vi "PSK_Packet_Transmit.vi"() -> ()   [LabVIEW 2014]
uses:
  <vilib>/Waveform/DWDTOps.llb/DWDT Analog to Digital.vi
  <vilib>/Waveform/DWDTOps.llb/DWDT Digital to Binary U8.vi
  <instrlib>/niUSRP/niUSRP Write Tx Data (CDB Cluster).vi
  <vilib>/Waveform/DWDTOps.llb/DWDT Binary U8 to Digital.vi
  <vilib>/Waveform/DWDTOps.llb/DWDT Digital to Analog.vi
  <vilib>/measure/NI_MABase.lvlib
panel:
  out "Array":i8[][](array[numeric])
  out "Waveform Graph":waveform(dbl)(graph)
  in  "phase":dbl format="%.2p"
  in  "sampling info":cluster{"Fs":dbl, "#s":dbl}={"Fs"=1000.0, "#s"=1000.0} {"Fs" format="%.2p"}
  out "error out":errorcluster
  in  "stop":bool
  in  "USRP IP address":refnum<k15>="192.168.10.2"
  in  "Tx Parameters":T1={"Tx IQ Sampling\nRate [s/sec]"=400000.0, "Tx Frequency [Hz]"=915000000.0, "Tx Gain [dB]"=0.0, "Tx Antenna"="TX1"} {"Tx Gain [dB]" format="%#.6p"; "Tx Frequency [Hz]" format="%#.6p"; "Tx IQ Sampling\nRate [s/sec]" format="%#.6p"}
  out "Actual Tx Parameters":T1={"Tx IQ Sampling\nRate [s/sec]"=400000.0, "Tx Frequency [Hz]"=915000000.0, "Tx Gain [dB]"=0.0, "Tx Antenna"="TX1"} {"Tx Gain [dB]" format="%#.6p"; "Tx Frequency [Hz]" format="%#.6p"; "Tx IQ Sampling\nRate [s/sec]" format="%#.6p"}
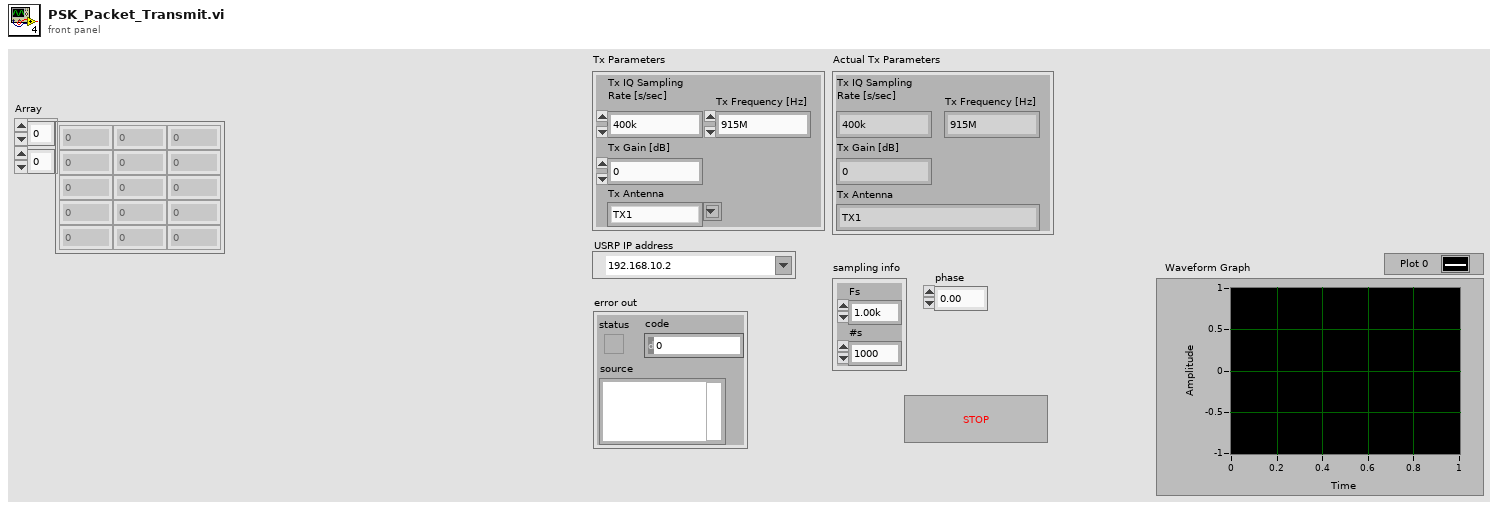
[diagram p1: front panel]
types:
  T1 = cluster{"Tx IQ Sampling\nRate [s/sec]":dbl, "Tx Frequency [Hz]":dbl, "Tx Gain [dB]":dbl, "Tx Antenna":string}
  T2 = typedef "niAMT.lvlib/Complex Data Waveform.ctl" = cluster{"t0":dbl, "dt":dbl, "Y":cdb[]}
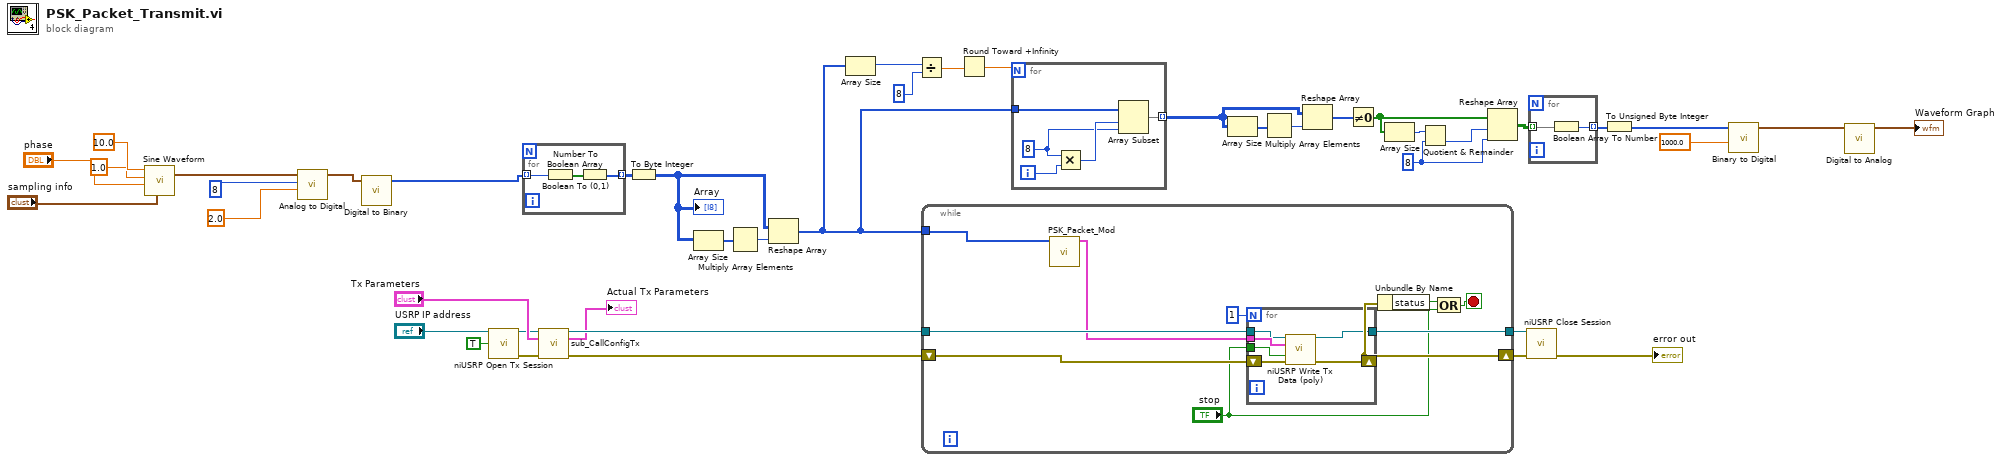
[diagram p0: block diagram]
diagram:
  w9 = 8 ("dimension size")
  n1 = call <vilib>:"Sine Waveform.vi"("sampling info"="sampling info", "phase"="phase", "amplitude"=1.0, "frequency"=10.0) -> ("signal out"=w32:waveform(dbl))  [unwired: 6 in, 1 out]
  n2 = call-poly <vilib>:"Analog to Digital.vi"("full-scale range (pk-pk)"=2.0, "resolution (16 bit)"=8, "analog waveform"=w32) -> ("digital waveform"=w25:digitalwaveform)  [unwired: 5 in, 3 out]
  n3 = call-poly <vilib>:"Digital to Binary.vi"("digital waveform"=w25) -> ("binary array"=w17:u8[])  [unwired: 9 in, 1 out]
  n4 = call <instrlib>:"niUSRP Open Tx Session.vi"("device names"="USRP IP address", "reset"=TRUE) -> ("session handle out"=w42:refnum<k15>, "error out"=w41:errorcluster)  [unwired: 12 in]
  n5 = for {
    tunnel: w17 -> [w46] mode=indexing
    tunnel: [w44] -> w21 mode=indexing
    n6 = Number To Boolean Array(number=w46) -> (Boolean array=w45:bool[])
    n7 = Boolean To (0,1)(Boolean=w45) -> (0, 1=w44:i16[])
  }
  n8 = call "sub_CallConfigTx.vi"("session handle"=w42, "Tx Parameters"="Tx Parameters", "error in"=w41) -> ("session handle out"=w36:refnum<k15>, "Actual Tx Parameters"=→"Actual Tx Parameters":T1, "error out"=w35:errorcluster)  [unwired: 10 in]
  n9 = To Byte Integer(number=w21) -> (8bit integer=w18:i8[][])
  "Array" <- w18
  n10 = Array Size(array=w18) -> (size(s)=w20:i32[])
  n11 = Multiply Array Elements(1:w20) -> (0:w19:i32)
  n12 = Reshape Array(w18, w19) -> (w12:i8[])
  n13 = Array Size(array=w12) -> (size(s)=w15:i32)
  n14 = Divide(x=w15, y=8) -> (x/y=w14:dbl)
  n15 = while {
    tunnel: w36 -> [w55]
    shift-right: [w52] -> w38
    shift-left: w35 -> [w56]
    tunnel: [w54] -> w37
    tunnel: w12 -> [w47]
    stop <- w51 stop-if-true
    n16 = call "PSK_Packet_Mod.vi"("user base bit pattern"=w47) -> ("output complex waveform"=w48:T2)  [unwired: 10 in]
    n17 = for {
      N: 1 -> [_]
      tunnel: w48 -> [w61]
      tunnel: w55 -> [w60]
      tunnel: [w59] -> w54
      tunnel: "stop" -> [w58]
      shift-right: [w57] -> w52
      shift-left: w56 -> [w62]
      n18 = call-poly <instrlib>:"niUSRP Write Tx Data (poly).vi"("session handle"=w60, "data"=w61, "end of data?"=w58, "error in (no error)"=w62) -> ("session handle out"=w59:refnum<k15>, "error out"=w57:errorcluster)  [unwired: 10 in]
    }
    n19 = Unbundle By Name(w52) -> ("status"=w53:bool)
    n20 = Compound Arithmetic op=OR(w53, "stop") -> (w51:bool)
  }
  n21 = Round Toward +Infinity(x=w14) -> (ceil(x): smallest int >= x=w13:dbl)
  n22 = for {
    N: w13 -> [_]
    tunnel: w12 -> [w67]
    tunnel: [w63] -> w1 mode=indexing
    i -> [w66]
    w64 = 8 ("x")
    n23 = Multiply(x=w64, y=w66) -> (x*y=w65:i32)
    n24 = Array Subset(array=w67, index=w65, length=w64) -> (w63:i8[])
  }
  n25 = Array Size(array=w1) -> (size(s)=w3:i32[])
  n26 = Multiply Array Elements(1:w3) -> (0:w4:i32)
  n27 = Reshape Array(w1, w4) -> (w2:i8[])
  n28 = Not Equal To 0?(x=w2) -> (x != 0?=w7:bool[])
  n29 = Array Size(array=w7) -> (size(s)=w8:i32)
  n30 = Quotient & Remainder(x=w8, y=w9) -> (floor(x/y)=w6:i32)  [unwired: 1 out]
  n31 = Reshape Array(w7, w6, w9) -> (w10:bool[][])
  n32 = call <instrlib>:"niUSRP Close Session.vi"("session handle"=w37, "error in (no error)"=w38) -> ("error out"=→"error out":errorcluster)  [unwired: 13 in]
  n33 = for {
    tunnel: w10 -> [w69] mode=indexing
    tunnel: [w68] -> w11 mode=indexing
    n34 = Boolean Array To Number(Boolean array=w69) -> (number=w68:u32)
  }
  n35 = To Unsigned Byte Integer(number=w11) -> (unsigned 8bit integer=w5:u8[])
  n36 = call-poly <vilib>:"Binary to Digital.vi"("sample rate"=1000.0, "binary array"=w5) -> ("digital waveform"=w22:digitalwaveform)  [unwired: 8 in, 1 out]
  n37 = call-poly <vilib>:"Digital to Analog.vi"("digital waveform"=w22) -> ("analog waveform"=→"Waveform Graph":waveform(dbl))  [unwired: 7 in, 3 out]
